vi "Cleanup.vi"(8 "error in (no error)":errorcluster, 11 "SerialConfigPanel in":refnum<class "SerialConfigPanel.lvclass">) -> (0 "error out":errorcluster)   [LabVIEW 2020, in "LV-Term.lvlib" / "SerialConfigPanel.lvclass"]
uses:
  SerialConfigPanel.lvclass
  SerialConfigPanel.lvclass/SerialConfigPanel.ctl
  <vilib>/IlluminatedG/IG OOPanel/OOPanel/Panel/Panel.lvclass
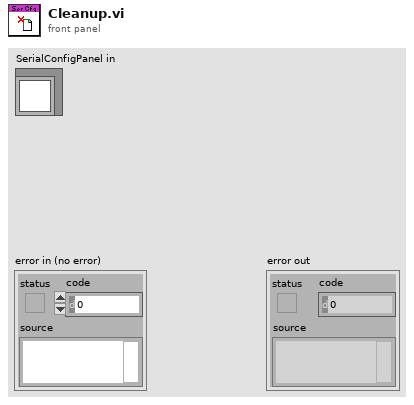
[diagram p1: front panel]
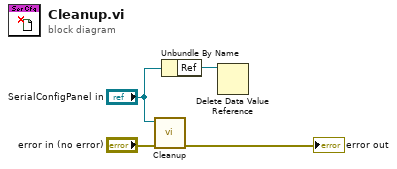
[diagram p0: block diagram]
diagram:
  n1 = call-parent "Cleanup.vi"("error in (no error)"="error in (no error)", "Panel in"="SerialConfigPanel in") -> ("error out"=→"error out":errorcluster)  [unwired: 9 in]
  n2 = Unbundle By Name("SerialConfigPanel in") -> ("Ref"=w2:refnum<data-value>)
  n3 = Delete Data Value Reference(data value reference=w2) -> ()  [unwired: 1 in, 2 out]
